vi "SP De-Embed Demo.vi"() -> ()   [LabVIEW 2011]
panel:
  in  "De-Embed 2":bool=TRUE
  in  "Orientation":string(combo)="Normal"
  in  "Port":string(combo)="1"
  in  "Check":bool
  in  "Serial":string="1" caption="Serial Number"
  in  "Model":string="SMA - N" caption="Model Number"
  in  "Devices":i32(listbox)
  in  "Check 4":bool
  in  "Check 3":bool
  in  "Check 2":bool
  in  "stop":bool
  in  "De-Embed":bool=TRUE
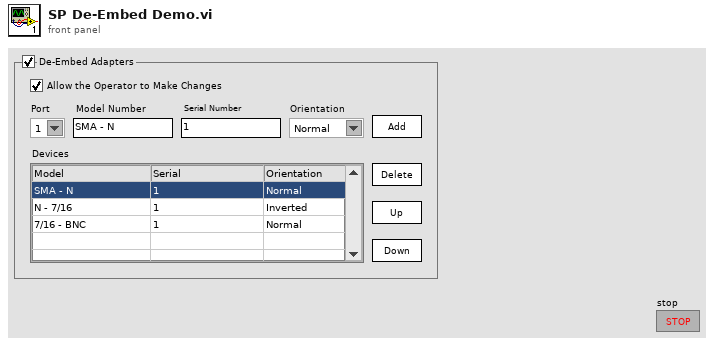
[diagram p1: front panel]
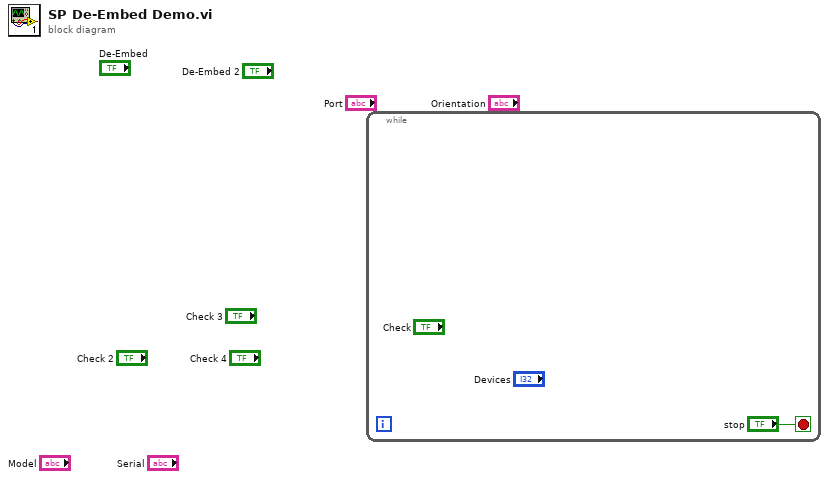
[diagram p0: block diagram]
diagram:
  n1 = while {
    stop <- "stop" stop-if-true
  }
